vi "send event info.vi"(7 "Type (Event)":T1(ring), 8 "error in":errorcluster, 10 "Info":string, 11 "node ref":T2) -> (0 "error out":errorcluster, 3 "node ref out":T2)   [LabVIEW 2020, in "Publisher Subscriber.lvlib"]
uses:
  Publisher Subscriber.lvlib
  Controls/event info.ctl
  Controls/data cluster.ctl
  Controls/subscription bank ref.ctl
  Controls/node dvr data.ctl
  Controls/node refnum.ctl
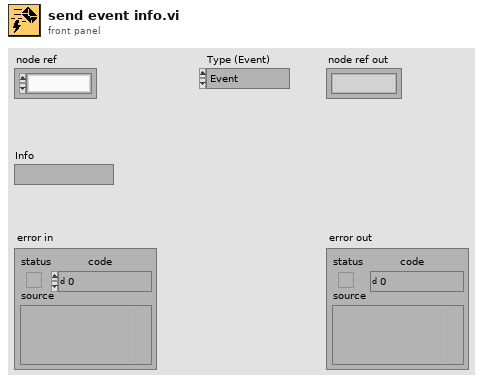
[diagram p1: front panel]
types:
  T1 = enum16{"Event", "Info", "Debug", "Warning", "Error"}
  T2 = typedef "Publisher Subscriber.lvlib/node refnum.ctl" = refnum<k1>
  T3 = typedef "Publisher Subscriber.lvlib/event info.ctl" = cluster{"Module Name":string, "Type":enum16{"Event", "Info", "Debug", "Warning", "Error"}, "Info":string}
  T4 = typedef "Publisher Subscriber.lvlib/node dvr data.ctl" = cluster{"queue ref":refnum<queue>, "Subscription Bank Ref":refnum<data-value>, "Command":string, "Data":variant, "Subscriptions []":set{string}, "Variables DVR Ref":refnum<data-value>}
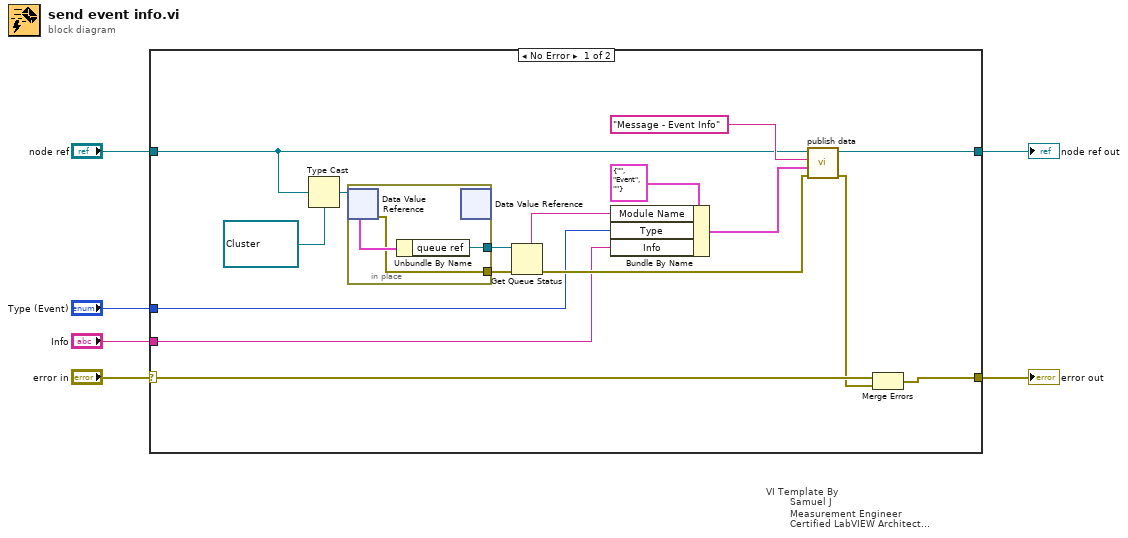
[diagram p0: block diagram]
diagram:
  n1 = case "VI Template By\n        Samuel J\n        Measurement Engineer\n        Certified LabVIEW Architect\n        Vestas Technology R&D Chennai" shown="No Error" "error in" {
    selector: "error in" -> [w18 w27]
    tunnel: [w12 w27] -> w5
    tunnel: "node ref" -> [w17 w26]
    tunnel: [w22 w26] -> w3
    tunnel: "Type (Event)" -> [w9 _]
    tunnel: "Info" -> [w8 _]
    frame No Error {
      n2 = Type Cast(type=refnum<data-value> refnum ("data value reference"), x=w17) -> (*(type *) &x=w16:refnum<data-value>)
      n3 = in-place {
        in-place-border: [w24] -> w15
        in-place-border: [w23] -> w10
        n4 = in-place-dvr #1(w16) -> (w25:T4, w23:errorcluster)
        n5 = Unbundle By Name(w25) -> ("queue ref"=w24:refnum<queue>)
        n6 = in-place-dvr #1() -> ()  [unwired: 1 in, 2 out]
      }
      n7 = Get Queue Status(queue=w15, error in (no error)=w10) -> (queue name=w14:string, error out=w13:errorcluster)  [unwired: 1 in, 6 out]
      n8 = Bundle By Name(cluster=T3 {"Module Name"="", "Type"=enum."Event", "Info"=""} ("error info"), "Module Name"=w14, "Type"=w9, "Info"=w8) -> (w20:T3)
      n9 = call "publish data.vi"("error in"=w13, "data in"=w20, "command"="Message - Event Info", "refnum in"=w17) -> ("error out"=w11:errorcluster, "refnum out"=w22:T2)  [unwired: 6 in]
      n10 = Merge Errors(w18, w11) -> (w12:errorcluster)
    }
    frame Error {
    }
  }
  "error out" <- w5
  "node ref out" <- w3
